vi "Dashboard Main.vi"() -> ()   [LabVIEW 2014]
uses:
  <vilib>/event_ctls.llb/eventvkey.ctl
  <vilib>/Rock Robotics/WPI/Dashboard/WPI_DashboardLogging Global.vi
  <vilib>/Utility/config.llb/Write Key (String).vi
  <vilib>/Utility/config.llb/Write Key (I32).vi
  <vilib>/Utility/config.llb/NI_LVConfig.lvlib
panel:
  in  "TCP":refnum<k5>
  in  "Rec Mode":enum32{"Stop", "Record", "Playback"}(radio)
  in  "Vision":u16(ring) items=["Camera Off", "USB Camera SW", "USB Camera HW", "IP Camera"]
  out "Camera IP":string
  out "Image Message":string="Timeout in Camera Communications"
  in  "Dashboard Tab":T1(tab)
  in  "Camera Settings":T2={"Frame Rate"=30, "Compression"=30, "Size"=1} {"Frame Rate" scale=1.0..30.0; "Size" items=["640x480", "320x240", "160x120"]}
  out "MotorChart R":cluster{"Numeric":dbl, "Numeric":dbl}(graph)
  out "MotorChart L":T3(graph)
  out "MotorSliders R":cluster{"MotorSlide1":dbl, "MotorSlide2":dbl} {"MotorSlide2" scale=-1.0..1.0 scale format="%#_2e"; "MotorSlide1" scale=-1.0..1.0 scale format="%#_2e"}
  out "MotorSliders L":T4 {"MotorSlide4 2" scale=0.0..14.0 scale format="%#_2e"; "MotorSlide2" scale=-1.0..1.0 scale format="%#_2e"; "MotorSlide1" scale=-1.0..1.0 scale format="%#_2e"}
  out "Gyro":dbl(knob) scale=0.0..360.0
  out "JS1 Z":dbl(slide) scale=-1.0..1.0 scale format="%#_2e"
  out "JS1 Graph":cluster{"X":dbl, "Y":dbl}[](graph)
  out "JS1 Buttons":T5
  out "JS2 Z":dbl(slide) scale=-1.0..1.0 scale format="%#_2e"
  out "JS2 Graph":cluster{"X":dbl, "Y":dbl}[](graph)
  out "JS2 Buttons":T5
  out "Mode":T6(ring)=enum."Auto Disabled"
  in  "DB Camera Config":bool
  out "fps":dbl format="%#.1g"
  out "Mbps":dbl format="%#.1g"
  out "Mbps 2":bool
  in  "DB/String 9":string
  in  "DB/String 8":string
  in  "DB/String 7":string
  in  "DB/String 6":string
  in  "DB/String 5":string
  in  "DB/String 4":string
  in  "DB/String 3":string
  in  "DB/String 2":string
  in  "DB/String 1":string
  in  "DB/String 0":string
  in  "DB/Slider 0":dbl(slide) scale=0.0..5.0
  in  "DB/Slider 1":dbl(slide) scale=0.0..5.0
  in  "DB/Slider 2":dbl(slide) scale=0.0..5.0
  in  "DB/Slider 3":dbl(slide) scale=0.0..5.0
  out "DB/LED 3":bool
  out "DB/LED 2":bool
  out "DB/LED 1":bool
  out "DB/LED 0":bool
  in  "DB/Button 3":bool
  in  "DB/Button 2":bool
  in  "DB/Button 1":bool
  in  "DB/Button 0":bool caption="New Name"
  in  "Test Slider":dbl(slide) scale=0.0..100.0 scale format="%#_3g"
  in  "On/Off":bool caption="Solenoid"
  in  "Test Name":u16(ring) items=["Select the test to run...", "Example Test", "-------------------------------", "List of tests is built in robot code.", "Replace with your own automated tests."]
  in  "Test Tree":string(tree)
  in  "Motor":cluster{"Value":dbl, "Enable":bool} {"Value" scale=-1.0..1.0 scale format="%#_3g"}
  out "Progress":T7 {"Test Progress" scale=0.0..100.0}
  in  "Rev/Fwd":cluster{"Forward":bool, "Reverse":bool}
  in  "Test Ring":u16(ring) items=["Monochrome", "Color"]
  in  "Listbox":i32(listbox)
  out "Tree":string(tree)
  out "Camera Image":T8(plugin-control)
  out "Boolean":bool
  # "Left"
  # "Front"
  # "Right"
  # "Battery"
  # "This tab is a great place for autonomous settings and robot-specific values.\nPlace controls and indicators inside this tab and match name to\nDashboard Variables on robot. You can also delete this comment."
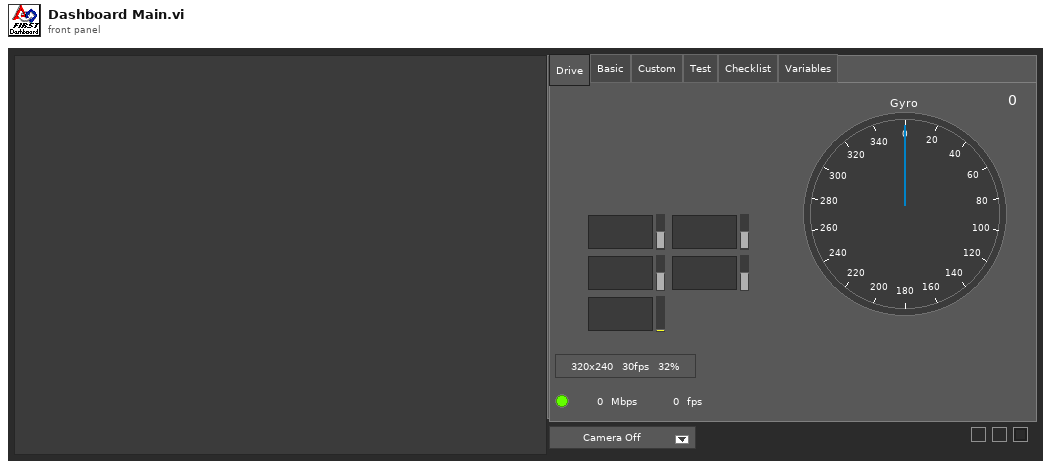
[diagram p1: front panel]
types:
  T1 = enum32{"Drive", "Basic", "Custom", "Test", "Checklist", "Variables"}
  T2 = cluster{"Frame Rate":i32, "Compression":i32, "Size":u16}
  T3 = cluster{"Numeric":dbl, "Numeric":dbl, "Battery V":dbl}
  T4 = cluster{"MotorSlide1":dbl, "MotorSlide2":dbl, "MotorSlide4 2":dbl}
  T5 = cluster{bool, bool, bool, bool, bool, bool, bool, bool, bool, bool, bool, bool}
  T6 = enum8{"Tele-Op Disabled", "Tele-Op Enabled", "Auto Disabled", "Auto Enabled", "Test Disabled", "Test Enabled", "Disconnected", "No Code", "E-Stop"}
  T7 = cluster{"Test Progress":u8, "Test Progress Text":string}
  T8 = typedef "IMAQ Image.ctl" = refnum<image>
  T9 = typedef "Image Type" = u32
  T10 = cluster{"Camera Image":refnum<vi>, "Dashboard Tab":refnum<vi>, "Boolean":refnum<vi>, "Vision":refnum<vi>, "Rec Mode":refnum<vi>, "Test Slider":refnum<vi>, "On/Off ":refnum<vi>, "Test Ring":refnum<vi>, "Rev/Fwd":refnum<vi>, "Test Name":refnum<vi>, "Motor":refnum<vi>, "Progress":refnum<vi>, "CheckList":refnum<vi>, "Tree":refnum<vi>, "Test Tree":refnum<vi>}
  T11 = cluster{"Error Strings":string, "Disable Counts":cluster{u16, u16}, "Rail Faults":cluster{u16, u16, u16}, "Robot IP":string, "DB Mode":u8, "Event Info":cluster{"Name":string, "Type":u8, "Number":u16, "Replay":u8}, "Camera Addr":string}
  T12 = cluster{"Storage":cluster{"Disk Free":u64, "RAM Block":u32, "RAM free":u32}, "CPU Utilization":cluster{"CPU % ISR":sgl, "CPU % Time Crit":sgl, "CPU % Timed Str":sgl, "CPU % High":sgl, "CPU % Above":sgl, "CPU % Normal":sgl, "CPU % Low":sgl}, "CAN":cluster{"% Bus Utilization":sgl, "Bus Off Cnt":u32, "TX_FIFO Full Cnt":u32, "Receive Error Cnt":u8, "Transmit Error Cnt":u8}, "HID":cluster{"HID Outputs":u32, "Rumble Low":u16, "Rumble High":u16}[]}
  T13 = cluster{"Status bits":cluster{"Test Mode":bool, "Autonomous":bool, "Enabled":bool, "Code Start":bool, "Brownout":bool, "Reserved 2":bool, "Reserved 3":bool, "E-Stop":bool}, "Code Trace":cluster{"Disabled":bool, "TeleOp":bool, "Auto":bool, "Test":bool}, "Controller Type":enum16{"unknown", "cRIO", "roboRio"}, "Code?":enum16{"unknown", "noCode", "code"}, "Battery V":dbl}
  T14 = cluster{"Control Bits":cluster{"TestMode":bool, "Autonomous":bool, "Enabled":bool, "FMS Present":bool, bool, bool, bool, "E-Stop":bool}, "Team Station ":u8, "Countdown":sgl, "Joystick Values":cluster{"Axes":dbl[], "Buttons":bool[], "POVs":i16[]}[]}
  T15 = cluster{"Axes":dbl[], "Buttons":bool[], "POVs":i16[]}[]
  T16 = cluster{"Axes":dbl[], "Buttons":bool[], "POVs":i16[]}
  T17 = cluster{"Buttons[0]":bool, "Buttons[1]":bool, "Buttons[2]":bool, "Buttons[3]":bool, "Buttons[4]":bool, "Buttons[5]":bool, "Buttons[6]":bool, "Buttons[7]":bool, "Buttons[8]":bool, "Buttons[9]":bool, "Buttons[10]":bool, "Buttons[11]":bool}
  T18 = typedef "NI_LVConfig.lvlib/Config Data RefNum.ctl" = refnum<k1>
  T19 = cluster{"Operation":enum16{"Update", "Clear"}, "Color Box":u32}[]
  T20 = typedef "eventvkey.ctl" = enum16{"ASCII", "Enter", "Return", "Shift", "Ctrl", "Alt", "Cmd", "Opt", "Caps", "NumLock", "Clear", "Break", "Up", "Down", "Left", "Right", "Insert", "Delete", "Home", "End", "PageUp", "PageDown", "Escape", "Help", "Pause", "ScrollLock", "F1", "F2", "F3", "F4", "F5", "F6", "F7", "F8", "F9", "F10", "F11", "F12", "F13", "F14", "F15", "F16", "F17", "F18", "F19", "F20", "F21", "F22", "F23", "F24", "Play", "VolumeUp", "VolumeDown", "Mute", "Two Byte Char"}
  T21 = cluster{"Image Size":bool, "Image Type":bool, "Pixel Value":bool, "ROI Information":bool, "Zoom Factor":bool}
  T22 = enum8{"Enabled", "Disabled", "Disabled and Grayed Out"}
  T23 = cluster{"Operation":enum16{"Update", "Clear"}, "Color Box":u32}
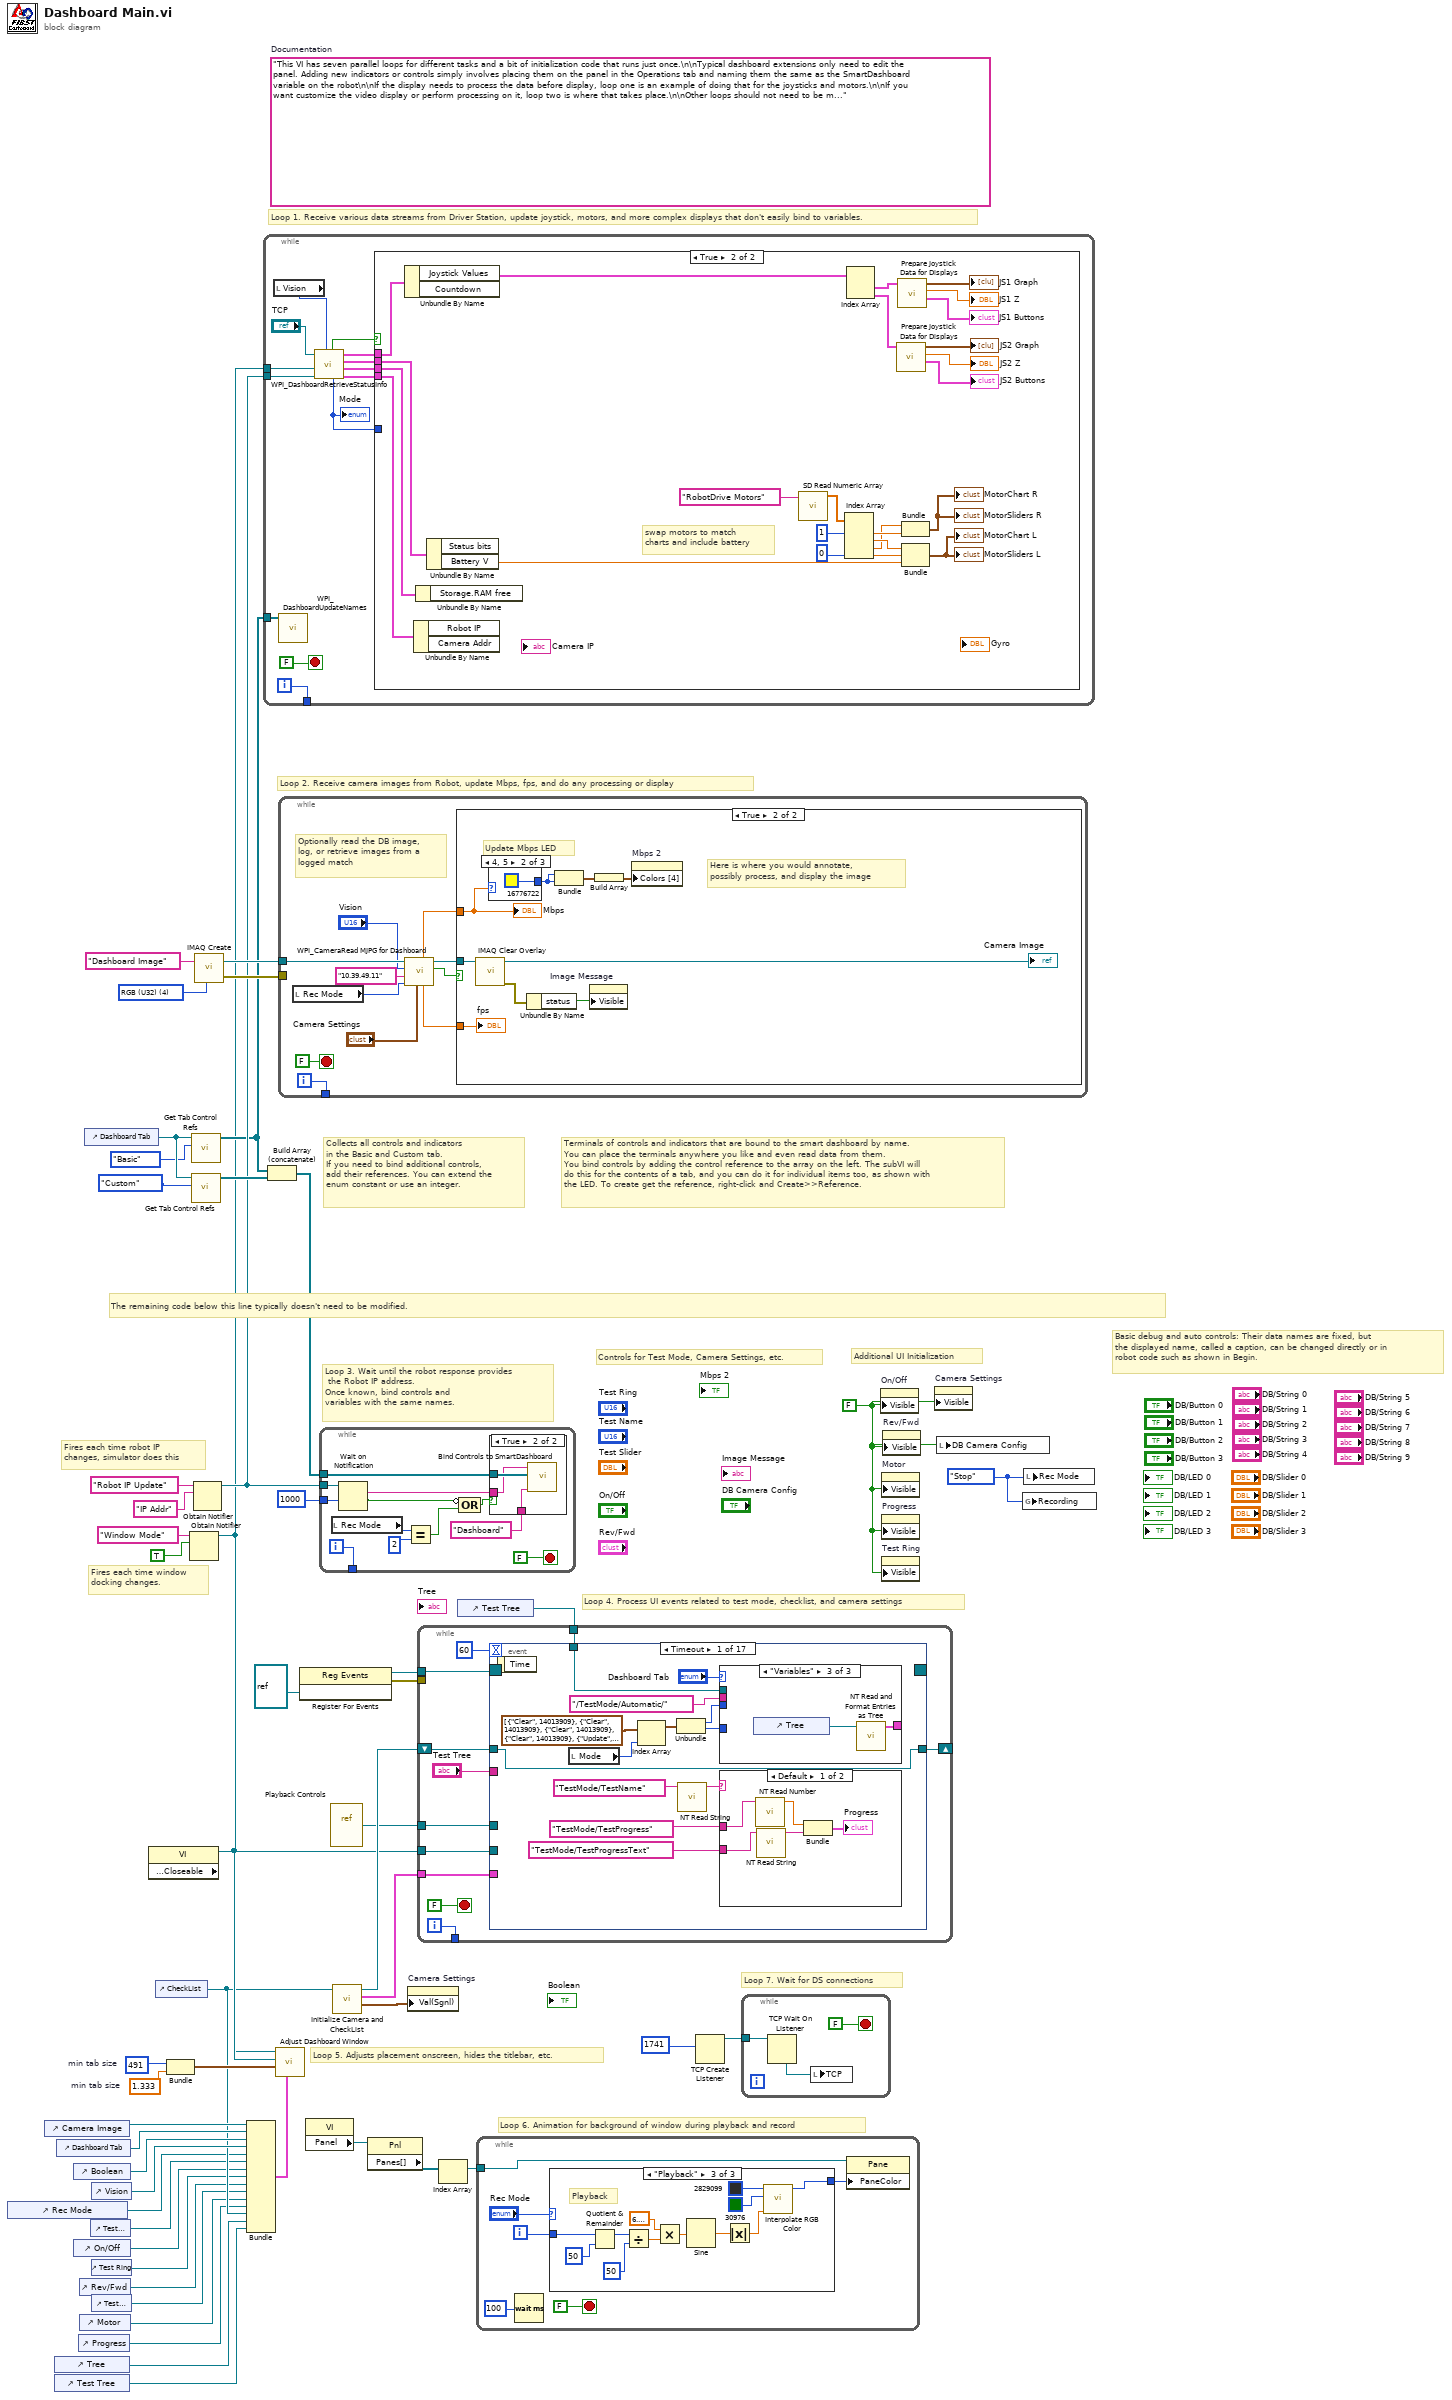
[diagram p0: block diagram]
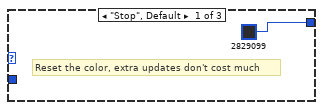
[diagram p3: hidden frame]
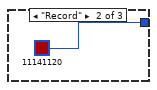
[diagram p4: hidden frame]
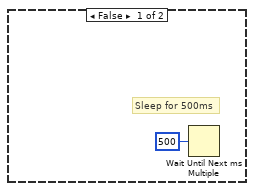
[diagram p6: hidden frame]
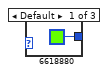
[diagram p7: hidden frame]
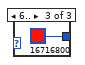
[diagram p8: hidden frame]
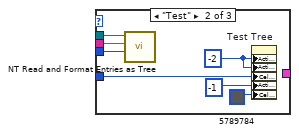
[diagram p10: hidden frame]
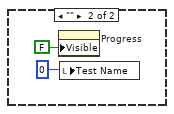
[diagram p11: hidden frame]
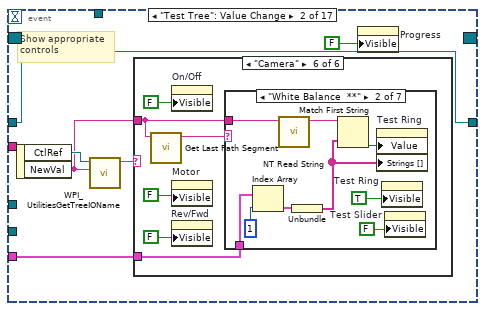
[diagram p12: hidden frame]
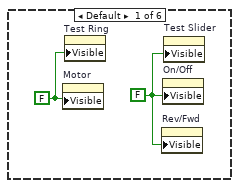
[diagram p13: hidden frame]
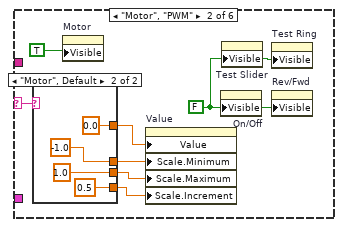
[diagram p14: hidden frame]
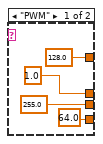
[diagram p15: hidden frame]
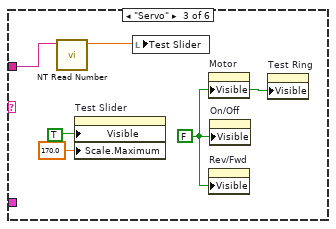
[diagram p16: hidden frame]
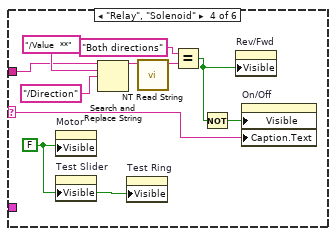
[diagram p17: hidden frame]
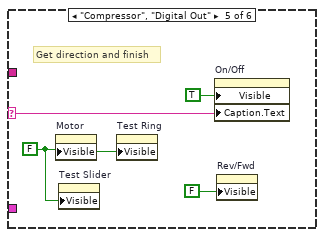
[diagram p18: hidden frame]
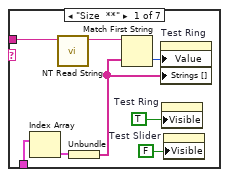
[diagram p19: hidden frame]
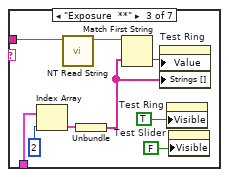
[diagram p20: hidden frame]
diagram:
  w24 = 491  # min tab size
  w23 = 1.333  # min tab size
  w32 = enum32{"Stop", "Record", "Playback"}."Stop" ("Rec Mode")
  w6 = FALSE ("Visible")
  (unwired) "This VI has seven parallel loops for different tasks and a bit of initialization code that runs just once.\n\nTypical dashboard extensions only need to edit the panel. Adding new indicators or controls simply involves placing them on the panel in the Operations tab and naming them the same as the SmartDashboard variable on the robot\n\nIf the display needs to process the data before display, loop one is an example of doing that for the joysticks and motors.\n\nIf you want customize the video display or perform processing on it, loop two is where that takes place.\n\nOther loops should not need to be modified. They are pretty standard, and document the task they perform."  # Documentation
  w52 = T9 4 items=["Grayscale (U8)", "Grayscale (I16)", "Grayscale (SGL)", "Complex (CSG)", "RGB (U32)", "HSL (U32)", "RGB (U64)"] ("Image Type")
  # "Loop 7. Wait for DS connections"
  # "Basic debug and auto controls: Their data names are fixed, but\nthe displayed name, called a caption, can be changed directly or in\nrobot code such as shown in Begin."
  # "Controls for Test Mode, Camera Settings, etc."
  # "Additional UI Initialization"
  # "Loop 6. Animation for background of window during playback and record"
  # "Fires each time robot IP\nchanges, simulator does this"
  # "Fires each time window\ndocking changes."
  # "Collects all controls and indicators\nin the Basic and Custom tab.\nIf you need to bind additional controls,\nadd their references. You can extend the\nenum constant or use an integer."
  # "The remaining code below this line typically doesn't need to be modified."
  # "Loop 4. Process UI events related to test mode, checklist, and camera settings"
  # "Terminals of controls and indicators that are bound to the smart dashboard by name.\nYou can place the terminals anywhere you like and even read data from them.\nYou bind controls by adding the control reference to the array on the left. The subVI will\ndo this for the contents of a tab, and you can do it for individual items too, as shown with\nthe LED. To create get the reference, right-click and Create>>Reference."
  # "Loop 3. Wait until the robot response provides\n the Robot IP address.\nOnce known, bind controls and\nvariables with the same names."
  # "Loop 5. Adjusts placement onscreen, hides the titlebar, etc."
  # "Loop 1. Receive various data streams from Driver Station, update joystick, motors, and more complex displays that don't easily bind to variables."
  # "Loop 2. Receive camera images from Robot, update Mbps, fps, and do any processing or display"
  n1 = control-ref of="Rec Mode"() -> (w12:refnum<vi>)
  n2 = control-ref of="Camera Image"() -> (w27:refnum<vi>)
  n3 = control-ref of="Tree"() -> (w16:refnum<vi>)
  n4 = control-ref of="Test Tree"() -> (w15:refnum<vi>)
  n5 = control-ref of="Dashboard Tab"() -> (w26:refnum<vi>)
  n6 = control-ref of="Boolean"() -> (w21:refnum<vi>)
  n7 = control-ref of="On/Off"() -> (w10:refnum<vi>)
  n8 = control-ref of="Progress"() -> (w7:refnum<vi>)
  n9 = control-ref of="Rev/Fwd"() -> (w8:refnum<vi>)
  n10 = control-ref of="Motor"() -> (w13:refnum<vi>)
  n11 = control-ref of="Dashboard Tab"() -> (w30:refnum<vi>)
  n12 = control-ref of="Test Slider"() -> (w11:refnum<vi>)
  n13 = control-ref of="Vision"() -> (w25:refnum<vi>)
  n14 = control-ref of="Test Ring"() -> (w9:refnum<vi>)
  n15 = control-ref of="Test Name"() -> (w14:refnum<vi>)
  n16 = property class="VI" props=["Front Panel.Closeable"]() -> (reference out=w31:refnum<vi>)  [unwired: 2 in, 2 out]
  n17 = control-ref of="CheckList"() -> (w17:refnum<vi>)
  n18 = Bundle("min tab size"=w24, "min tab size"=w23) -> (w22:cluster{"min tab size":i32, "min tab size":dbl})  [unwired: 1 in]
  n19 = Obtain Notifier(name (unnamed)="Window Mode", notification data type=TRUE) -> (notifier out=w3:refnum<notifier>)  [unwired: 2 in, 2 out]
  n20 = call <vilib>:"Get Tab Control Refs.vi"("Page Index"=T1."Basic" ("Dashboard Tab"), "TabControl in"=w30) -> ("ControlsOnPage"=w4:refnum<vi>[])  [unwired: 9 in]
  n21 = call <vilib>:"Get Tab Control Refs.vi"("Page Index"=T1."Custom" ("Dashboard Tab"), "TabControl in"=w30) -> ("ControlsOnPage"=w29:refnum<vi>[])  [unwired: 9 in]
  n22 = Obtain Notifier(name (unnamed)="Robot IP Update", notification data type="IP Addr" ("name (unnamed)")) -> (notifier out=w5:refnum<notifier>)  [unwired: 2 in, 2 out]
  n23 = call "IMAQ Create"("Image Name"="Dashboard Image", "Image Type"=w52) -> ("New Image"=w50:T8, "error out"=w49:errorcluster)  [unwired: 2 in, 1 out]
  n24 = Bundle("Camera Image"=w27, "Dashboard Tab"=w26, "Boolean"=w21, "Vision"=w25, "Rec Mode"=w12, "Test Slider"=w11, "On/Off"=w10, "Test Ring"=w9, "Rev/Fwd"=w8, "Test Name"=w14, "Motor"=w13, "Progress"=w7, "CheckList"=w17, "Tree"=w16, "Test Tree"=w15) -> (w18:T10)  [unwired: 1 in]
  n25 = while {
    tunnel: [w64] -> _
    tunnel: w5 -> [w58]
    tunnel: w4 -> [w57]
    tunnel: w3 -> [w53]
    i -> [w64]
    stop <- FALSE stop-if-true
    n26 = local read "Vision"() -> (w55:u16)
    n27 = call <vilib>:"WPI_DashboardUpdateNames.vi"("Controls on Tab"=w57) -> ()  [unwired: 11 in]
    n28 = call <vilib>:"WPI_DashboardRetrieveStatusInfo.vi"("Vision"=w55, "Binding Refnum"=w58, "Window Mode Notifier"=w53, "TCP Cnx"="TCP") -> ("Power and Errors"=w59:T11, "Robot Metrics"=w62:T12, "Status Info"=w63:T13, "Control Info"=w60:T14, "Robot Mode"=w56:T6, "Process?"=w61:bool)  [unwired: 2 in]
    "Mode" <- w56
    n29 = case shown="True" w61 {
      tunnel: w63 -> [_ w89]
      tunnel: w62 -> [_ w88]
      tunnel: w60 -> [_ w87]
      tunnel: w59 -> [_ w86]
      tunnel: w56 -> [_ _]
      frame False {
      }
      frame True {
        # "swap motors to match\ncharts and include battery"
        n30 = Unbundle By Name(w87) -> ("Joystick Values"=w74:T15)  [unwired: 1 out]
        n31 = Unbundle By Name(w86) -> ()  [unwired: 2 out]
        n32 = Unbundle By Name(w88) -> ()  [unwired: 1 out]
        n33 = Unbundle By Name(w89) -> ("Battery V"=w75:dbl)  [unwired: 1 out]
        n34 = call <vilib>:"SD Read Numeric Array.vi"("Name"="RobotDrive Motors") -> ("Numeric Array"=w77:dbl[])  [unwired: 8 in, 2 out]
        n35 = Index Array(array=w77, index #1=1, index #4=0) -> (element #1=w81:dbl, element #2=w82:dbl, element #3=w80:dbl, element #4=w85:dbl)  [unwired: 2 in]
        n36 = Index Array(array=w74) -> (element #1=w73:T16, element #2=w69:T16)  [unwired: 2 in]
        n37 = call "Prepare Joystick Data for Displays.vi"("Joystick Values"=w69) -> ("Buttons"=→"JS2 Buttons":T17, "Z Axis"=→"JS2 Z":dbl, "Cartesian Data"=→"JS2 Graph":cluster{"X axis":dbl, "X axis":dbl}[])  [unwired: 8 in]
        n38 = call "Prepare Joystick Data for Displays.vi"("Joystick Values"=w73) -> ("Buttons"=→"JS1 Buttons":T17, "Z Axis"=→"JS1 Z":dbl, "Cartesian Data"=→"JS1 Graph":cluster{"X axis":dbl, "X axis":dbl}[])  [unwired: 8 in]
        n39 = Bundle("Numeric"=w80, "Numeric"=w81) -> (→"MotorChart R" →"MotorSliders R":cluster{"Numeric":dbl, "Numeric":dbl})  [unwired: 1 in]
        n40 = Bundle("Numeric"=w82, "Numeric"=w85, "Battery V"=w75) -> (→"MotorChart L" →"MotorSliders L":T3)  [unwired: 1 in]
      }
    }
  }
  n41 = Build Array (concatenate)(w4, w29) -> (w28:refnum<vi>[])
  n42 = call "Adjust Dashboard Window.vi"("Sizing Refnums"=w18, "Size Constraints"=w22, "VI"=w31, "Notifier in"=w3) -> ()  [unwired: 8 in]
  n43 = while {
    tunnel: w50 -> [w98]
    tunnel: w49 -> [_]
    tunnel: [w99] -> _
    i -> [w99]
    stop <- FALSE stop-if-true
    # "Optionally read the DB image,\nlog, or retrieve images from a\nlogged match"
    n44 = local read "Rec Mode"() -> (w92:enum32{"Stop", "Record", "Playback"})
    n45 = call <vilib>:"WPI_CameraRead MJPG for Dashboard.vi"("Camera Settings"="Camera Settings", "Rec Mode"=w92, "Camera IP"="10.39.49.11", "Camera Mode"="Vision", "Refnum in"=w98) -> ("Active"=w96:bool, "Refnum out"=w97:T8, "FPS"=w95:dbl, "Bandwidth (Mbps)"=w94:dbl)  [unwired: 3 in]
    n46 = case shown="True" w96 {
      tunnel: w97 -> [_ w105]
      tunnel: w94 -> [_ w104]
      tunnel: w95 -> [_ w102]
      frame False {
        # "Sleep for 500ms"
        n47 = Wait Until Next ms Multiple(millisecond multiple=u32 500) -> ()  [unwired: 1 out]
      }
      frame True {
        # "Here is where you would annotate,\npossibly process, and display the image"
        # "Update Mbps LED"
        n48 = call "IMAQ Clear Overlay"("Image"=w105) -> ("error out"=w109:errorcluster, "Image Out"=→"Camera Image":T8)  [unwired: 2 in, 7 out]
        n49 = case shown="4, 5" w104 {
          tunnel: [u32 6618880 ("Color Box") u32 16776722 ("Color Box") u32 16716800 ("Color Box")] -> w106
          frame Default {
          }
          frame 4, 5 {
          }
          frame 6.. {
          }
        }
        n50 = Unbundle By Name(w109) -> ("status"=w110:bool)
        n51 = Bundle("Color Box"=w106, "Color Box"=w106) -> (w108:cluster{"Color Box":u32, "Color Box":u32})  [unwired: 1 out]
        n52 = property on="Image Message" class="Str"("Visible"=w110) -> ()  [unwired: 2 in, 2 out]
        n53 = Build Array(w108) -> (w107:cluster{"Color Box":u32, "Color Box":u32}[])
        n54 = property on="Mbps 2" class="Bool (strict)"("Colors [4]"=w107) -> ()  [unwired: 2 in, 2 out]
        "Mbps" <- w104
        "fps" <- w102
      }
    }
  }
  n55 = register-events(refnum<vi> refnum) -> (reference out=w36:refnum<event-registration>, error out=w35:errorcluster)  [unwired: 2 in]
  n56 = property class="VI"() -> ("Panel"=w39:refnum<vi>)  [unwired: 2 in, 2 out]
  n57 = while {
    tunnel: w28 -> [w125]
    tunnel: w5 -> [w123]
    tunnel: [w121] -> _
    tunnel: u32 1000 ("milliseconds to wait") -> [w120]
    i -> [w121]
    stop <- FALSE stop-if-true
    n58 = local read "Rec Mode"() -> (w116:enum32{"Stop", "Record", "Playback"})
    n59 = Wait on Notification(notifier=w123, timeout in ms (-1)=w120) -> (notification=w122:string, timed out?=w118:bool)  [unwired: 2 in, 2 out]
    n60 = Equal?(x=w116, y=u16 2 ("Rec Mode")) -> (x = y?=w117:bool)
    n61 = Compound Arithmetic op=OR(invert w118, w117) -> (w119:bool)
    n62 = case shown="True" w119 {
      tunnel: w125 -> [_ w128]
      tunnel: w122 -> [_ w127]
      tunnel: "Dashboard" -> [_ w126]
      frame False {
      }
      frame True {
        n63 = call <vilib>:"Bind Controls to SmartDashboard.vi"("Client Name"=w126, "Bound Control Refs"=w128, "Server IP Address"=w127) -> ()  [unwired: 9 in]
      }
    }
  }
  n64 = vi-ref "Playback Controls.vi"() -> (w37:refnum<vi>)
  n65 = call "Initialize Camera and CheckList.vi"("ListBox in"=w17) -> ("Cluster"=w43:cluster{"value":i32, "value":i32, "index":i32}, "Array"=w44:cluster{string[]}[], "File Refnum"=w42:T18)  [unwired: 8 in]
  n66 = property class="Pnl"(reference=w39) -> ("Panes[]"=w40:refnum<vi>[])  [unwired: 1 in, 2 out]
  n67 = property on="Camera Settings" class="Clust (strict)"("Val(Sgnl)"=w43) -> ()  [unwired: 2 in, 2 out]
  n68 = Index Array(array=w40) -> (element=w38:refnum<vi>)  [unwired: 1 in]
  n69 = control-ref of="Test Tree"() -> (w41:refnum<vi>)
  n70 = while {
    tunnel: w44 -> [w136]
    shift-right: [w135] -> _
    shift-left: w42 -> [w134]
    tunnel: [w133] -> _
    tunnel: w41 -> [w132]
    tunnel: w37 -> [w131]
    tunnel: w36 -> [w130]
    tunnel: w35 -> [_]
    tunnel: w31 -> [w129]
    i -> [w133]
    stop <- FALSE stop-if-true
    n71 = event shown="[0] Timeout" {
      selector: w130 -> [_ _ _ _ _ _ _ _ _ _ _ _ _ _ _ _ _]
      dyn-events: [_ _ _ _ _ _ _ _ _ _ _ _ _ w374 _ _ _] -> _
      timeout: u32 60 ("milliseconds to wait") -> [_ _ _ _ _ _ _ _ _ _ _ _ _ _ _ _ _]
      tunnel: w132 -> [w148 _ _ _ _ _ _ _ _ _ _ _ _ _ _ _ _]
      tunnel: "Test Tree" -> [_ _ _ _ _ _ _ _ w343 w351 w353 w357 w365 _ _ _ _]
      tunnel: w136 -> [_ w170 _ _ _ _ w307 w337 _ _ _ _ _ _ _ _ _]
      tunnel: [w144 w169 w268 w273 w281 w293 w306 w330 w342 w349 w352 w356 w364 w376 w390 w391 w401] -> w135
      tunnel: w134 -> [w144 w169 w268 w273 w281 w293 w305 w330 w342 w349 w352 w356 w364 w376 w390 w391 w401]
      tunnel: w131 -> [_ _ _ _ _ _ _ _ _ _ _ _ _ w377 _ w394 _]
      tunnel: w129 -> [_ _ _ _ _ _ _ _ _ _ _ _ _ w372 _ _ _]
      event Timeout {
        n72 = event-data() -> ()  [unwired: 1 in, 1 out]
        n73 = local read "Mode"() -> (w147:T6)
        n74 = Index Array(array=T19 [{"Operation"=enum."Clear", "Color Box"=14013909}, {"Operation"=enum."Clear", "Color Box"=14013909}, {"Operation"=enum."Clear", "Color Box"=14013909}, {"Operation"=enum."Clear", "Color Box"=14013909}, {"Operation"=enum."Update", "Color Box"=14013909}, {"Operation"=enum."Update", "Color Box"=16777215}, {"Operation"=enum."Clear", "Color Box"=14013909}, {"Operation"=enum."Clear", "Color Box"=14013909}, {"Operation"=enum."Clear", "Color Box"=14013909}], index=w147) -> (element=w142:T23)
        n75 = Unbundle(w142) -> ("Operation"=w141:enum16{"Update", "Clear"}, "Color Box"=w140:u32)
        n76 = call <vilib>:"NT Read String.vi"("Name"="TestMode/TestName") -> ("String"=w151:string)  [unwired: 9 in, 1 out]
        n77 = case shown="\"Variables\"" "Dashboard Tab" {
          tunnel: w148 -> [_ w159 _]
          tunnel: "/TestMode/Automatic/" ("Name Pattern") -> [_ w158 _]
          tunnel: w141 -> [_ w157 _]
          tunnel: [_ _ w161] -> _
          tunnel: w140 -> [_ w153 _]
          frame "Custom", Default {
          }
          frame "Test" {
            w156 = -2 ("Active Item:Row Number")
            n78 = call <vilib>:"NT Read and Format Entries as Tree.vi"("Operation"=w157, "Name Pattern"=w158, "Tree Refnum"=w159) -> ()  [unwired: 7 in, 2 out]
            n79 = property on="Test Tree" class="Tree (strict)"("Active Item Row Number"=w156, "ActiveColNum"=w156, "CellBG"=w153, "Active Item Row Number"=-1 ("Active Item:Row Number"), "CellBG"=u32 5789784 ("Color Box")) -> ()  [unwired: 2 in, 2 out]
          }
          frame "Variables" {
            n80 = control-ref of="Tree"() -> (w160:refnum<vi>)
            n81 = call <vilib>:"NT Read and Format Entries as Tree.vi"("Tree Refnum"=w160) -> ("Formatted Strings"=w161:cluster{"Name":string, "Value":string}[])  [unwired: 9 in, 1 out]
          }
        }
        n82 = case shown="Default" w151 {
          tunnel: "TestMode/TestProgress" ("Name") -> [w163 _]
          tunnel: "TestMode/TestProgressText" ("Name") -> [w162 _]
          frame Default {
            n83 = call <vilib>:"NT Read Number.vi"("Name"=w163) -> ("Numeric"=w164:dbl)  [unwired: 9 in, 1 out]
            n84 = call <vilib>:"NT Read String.vi"("Name"=w162) -> ("String"=w165:string)  [unwired: 9 in, 1 out]
            n85 = Bundle("Numeric"=w164, "String"=w165) -> (→"Progress":cluster{"Numeric":dbl, "String":string})  [unwired: 1 in]
          }
          frame "" {
            n86 = property on="Progress" class="Clust (strict)"("Visible"=FALSE) -> ()  [unwired: 2 in, 2 out]
            n87 = local write "Test Name"(u16 0) -> ()
          }
        }
      }
      event "Test Tree": Value Change {
        # "Show appropriate\ncontrols"
        n88 = event-data() -> ("CtlRef"=w173:refnum<vi>, "NewVal"=w171:string)  [unwired: 1 in]
        n89 = call <vilib>:"WPI_UtilitiesGetTreeIOName.vi"("NewVal"=w171, "TreeControl in"=w173) -> ("I/O Name"=w174:string)  [unwired: 9 in]
        n90 = case shown="\"Camera\"" w174 {
          selector: w174 -> [_ w181 _ w199 w208 _]
          tunnel: w171 -> [_ _ w196 w198 _ w215]
          tunnel: w170 -> [_ _ _ _ _ w214]
          frame Default {
            w176 = FALSE ("Visible")
            w175 = FALSE ("Visible")
            n91 = property on="Motor" class="Clust (strict)"("Visible"=w175) -> ()  [unwired: 2 in, 2 out]
            n92 = property on="Test Ring" class="Ring (strict)"("Visible"=w175) -> ()  [unwired: 2 in, 2 out]
            n93 = property on="Rev/Fwd" class="Clust (strict)"("Visible"=w176) -> ()  [unwired: 2 in, 2 out]
            n94 = property on="On/Off" class="Bool (strict)"("Visible"=w176) -> ()  [unwired: 2 in, 2 out]
            n95 = property on="Test Slider" class="Slide (strict)"("Visible"=w176) -> ()  [unwired: 2 in, 2 out]
          }
          frame "Motor", "PWM" {
            w182 = FALSE ("Visible")
            n96 = case shown="\"Motor\", Default" w181 {
              tunnel: [1.0 ("Value") -1.0 ("Value")] -> w180
              tunnel: [255.0 ("Value") 1.0 ("Value")] -> w179
              tunnel: [128.0 ("Value") 0.0 ("Value")] -> w178
              tunnel: [64.0 ("Value") 0.5 ("Value")] -> w177
              frame "PWM" {
              }
              frame "Motor", Default {
              }
            }
            n97 = property on="Motor" class="Clust (strict)"("Visible"=TRUE) -> ()  [unwired: 2 in, 2 out]
            n98 = property on="Value" class="Slide (strict)"("Value"=w178, "Scale.Minimum"=w180, "Scale.Maximum"=w179, "Scale.Increment"=w177) -> ()  [unwired: 2 in, 2 out]
            n99 = property on="On/Off" class="Bool (strict)"("Visible"=w182) -> ()  [unwired: 2 in, 2 out]
            n100 = property on="Test Slider" class="Slide (strict)"("Visible"=w182) -> ()  [unwired: 2 in, 2 out]
            n101 = property on="Test Ring" class="Ring (strict)"("Visible"=w182) -> ()  [unwired: 2 in, 2 out]
            n102 = property on="Rev/Fwd" class="Clust (strict)"("Visible"=w182) -> ()  [unwired: 2 in, 2 out]
          }
          frame "Servo" {
            w194 = FALSE ("Visible")
            n103 = call <vilib>:"NT Read Number.vi"("Name"=w196) -> ("Numeric"=w195:dbl)  [unwired: 9 in, 1 out]
            n104 = property on="Test Slider" class="Slide (strict)"("Visible"=TRUE, "Scale.Maximum"=170.0 ("Scale.Range:Maximum")) -> ()  [unwired: 2 in, 2 out]
            n105 = local write "Test Slider"(w195) -> ()
            n106 = property on="Motor" class="Clust (strict)"("Visible"=w194) -> ()  [unwired: 2 in, 2 out]
            n107 = property on="Rev/Fwd" class="Clust (strict)"("Visible"=w194) -> ()  [unwired: 2 in, 2 out]
            n108 = property on="On/Off" class="Bool (strict)"("Visible"=w194) -> ()  [unwired: 2 in, 2 out]
            n109 = property on="Test Ring" class="Ring (strict)"("Visible"=w194) -> ()  [unwired: 2 in, 2 out]
          }
          frame "Relay", "Solenoid" {
            w197 = FALSE ("Visible")
            n110 = property on="Motor" class="Clust (strict)"("Visible"=w197) -> ()  [unwired: 2 in, 2 out]
            n111 = property on="Test Slider" class="Slide (strict)"("Visible"=w197) -> ()  [unwired: 2 in, 2 out]
            n112 = Search and Replace String(input string=w198, search string="/Value  **", replace string="/Direction") -> (result string=w204:string)  [unwired: 5 in, 3 out]
            n113 = property on="Test Ring" class="Ring (strict)"("Visible"=w197) -> ()  [unwired: 2 in, 2 out]
            n114 = call <vilib>:"NT Read String.vi"("Name"=w204) -> ("String"=w202:string)  [unwired: 9 in, 1 out]
            n115 = Equal?(x="Both directions", y=w202) -> (x = y?=w200:bool)
            n116 = Not(x=w200) -> (.not. x?=w201:bool)
            n117 = property on="Rev/Fwd" class="Clust (strict)"("Visible"=w200) -> ()  [unwired: 2 in, 2 out]
            n118 = property on="On/Off" class="Bool (strict)"("Visible"=w201, "Caption.Text"=w199) -> ()  [unwired: 2 in, 2 out]
          }
          frame "Compressor", "Digital Out" {
            w207 = FALSE ("Visible")
            # "Get direction and finish"
            n119 = property on="Motor" class="Clust (strict)"("Visible"=w207) -> ()  [unwired: 2 in, 2 out]
            n120 = property on="Test Slider" class="Slide (strict)"("Visible"=w207) -> ()  [unwired: 2 in, 2 out]
            n121 = property on="Test Ring" class="Ring (strict)"("Visible"=w207) -> ()  [unwired: 2 in, 2 out]
            n122 = property on="On/Off" class="Bool (strict)"("Visible"=TRUE, "Caption.Text"=w208) -> ()  [unwired: 2 in, 2 out]
            n123 = property on="Rev/Fwd" class="Clust (strict)"("Visible"=FALSE) -> ()  [unwired: 2 in, 2 out]
          }
          frame "Camera" {
            n124 = call <vilib>:"Get Last Path Segment.vi"("String in"=w215) -> ("String out"=w216:string)  [unwired: 10 in]
            n125 = property on="On/Off" class="Bool (strict)"("Visible"=FALSE) -> ()  [unwired: 2 in, 2 out]
            n126 = property on="Motor" class="Clust (strict)"("Visible"=FALSE) -> ()  [unwired: 2 in, 2 out]
            n127 = property on="Rev/Fwd" class="Clust (strict)"("Visible"=FALSE) -> ()  [unwired: 2 in, 2 out]
            n128 = case shown="\"White Balance  **\"" w216 {
              tunnel: w215 -> [w222 w231 w240 w249 w258 _ w264]
              tunnel: w214 -> [w220 w228 w237 w246 w255 _ _]
              frame "Size  **" {
                n129 = Index Array(array=w220) -> (element=w219:cluster{string[]})  [unwired: 1 in]
                n130 = call <vilib>:"NT Read String.vi"("Name"=w222) -> ("String"=w221:string)  [unwired: 9 in, 1 out]
                n131 = Unbundle(w219) -> (w217:string[])
                n132 = Match First String(2:w217, 3:w221) -> (0:w218:i32)  [unwired: 1 out]
                n133 = property on="Test Ring" class="Ring (strict)"("Value"=w218, "Strings []"=w217) -> ()  [unwired: 2 in, 2 out]
                n134 = property on="Test Ring" class="Ring (strict)"("Visible"=TRUE) -> ()  [unwired: 2 in, 2 out]
                n135 = property on="Test Slider" class="Slide (strict)"("Visible"=FALSE) -> ()  [unwired: 2 in, 2 out]
              }
              frame "White Balance  **" {
                n136 = Index Array(array=w228, index=1) -> (element=w229:cluster{string[]})
                n137 = call <vilib>:"NT Read String.vi"("Name"=w231) -> ("String"=w230:string)  [unwired: 9 in, 1 out]
                n138 = Unbundle(w229) -> (w226:string[])
                n139 = Match First String(2:w226, 3:w230) -> (0:w225:i32)  [unwired: 1 out]
                n140 = property on="Test Ring" class="Ring (strict)"("Value"=w225, "Strings []"=w226) -> ()  [unwired: 2 in, 2 out]
                n141 = property on="Test Ring" class="Ring (strict)"("Visible"=TRUE) -> ()  [unwired: 2 in, 2 out]
                n142 = property on="Test Slider" class="Slide (strict)"("Visible"=FALSE) -> ()  [unwired: 2 in, 2 out]
              }
              frame "Exposure  **" {
                n143 = Index Array(array=w237, index=2) -> (element=w238:cluster{string[]})
                n144 = call <vilib>:"NT Read String.vi"("Name"=w240) -> ("String"=w239:string)  [unwired: 9 in, 1 out]
                n145 = Unbundle(w238) -> (w234:string[])
                n146 = Match First String(2:w234, 3:w239) -> (0:w235:i32)  [unwired: 1 out]
                n147 = property on="Test Ring" class="Ring (strict)"("Value"=w235, "Strings []"=w234) -> ()  [unwired: 2 in, 2 out]
                n148 = property on="Test Ring" class="Ring (strict)"("Visible"=TRUE) -> ()  [unwired: 2 in, 2 out]
                n149 = property on="Test Slider" class="Slide (strict)"("Visible"=FALSE) -> ()  [unwired: 2 in, 2 out]
              }
              frame "Exposure Priority  **" {
                n150 = Index Array(array=w246, index=3) -> (element=w247:cluster{string[]})
                n151 = call <vilib>:"NT Read String.vi"("Name"=w249) -> ("String"=w248:string)  [unwired: 9 in, 1 out]
                n152 = Unbundle(w247) -> (w243:string[])
                n153 = Match First String(2:w243, 3:w248) -> (0:w244:i32)  [unwired: 1 out]
                n154 = property on="Test Ring" class="Ring (strict)"("Value"=w244, "Strings []"=w243) -> ()  [unwired: 2 in, 2 out]
                n155 = property on="Test Ring" class="Ring (strict)"("Visible"=TRUE) -> ()  [unwired: 2 in, 2 out]
                n156 = property on="Test Slider" class="Slide (strict)"("Visible"=FALSE) -> ()  [unwired: 2 in, 2 out]
              }
              frame "Color Enable  **" {
                n157 = Index Array(array=w255, index=4) -> (element=w256:cluster{string[]})
                n158 = call <vilib>:"NT Read String.vi"("Name"=w258) -> ("String"=w257:string)  [unwired: 9 in, 1 out]
                n159 = Unbundle(w256) -> (w252:string[])
                n160 = Match First String(2:w252, 3:w257) -> (0:w253:i32)  [unwired: 1 out]
                n161 = property on="Test Ring" class="Ring (strict)"("Value"=w253, "Strings []"=w252) -> ()  [unwired: 2 in, 2 out]
                n162 = property on="Test Ring" class="Ring (strict)"("Visible"=TRUE) -> ()  [unwired: 2 in, 2 out]
                n163 = property on="Test Slider" class="Slide (strict)"("Visible"=FALSE) -> ()  [unwired: 2 in, 2 out]
              }
              frame Default {
                n164 = property on="Test Ring" class="Ring (strict)"("Visible"=FALSE) -> ()  [unwired: 2 in, 2 out]
                n165 = property on="Test Slider" class="Slide (strict)"("Visible"=FALSE) -> ()  [unwired: 2 in, 2 out]
              }
              frame "Brightness  **", "Color Level  **", "Compression  **", "FPS  **", "Sharpness  **" {
                n166 = call <vilib>:"NT Read Number.vi"("Name"=w264) -> ("Numeric"=w263:dbl)  [unwired: 9 in, 1 out]
                n167 = local write "Test Slider"(w263) -> ()
                n168 = property on="Test Slider" class="Slide (strict)"("Visible"=TRUE, "Scale.Maximum"=100.0 ("Scale.Range:Maximum")) -> ()  [unwired: 2 in, 2 out]
                n169 = property on="Test Ring" class="Ring (strict)"("Visible"=FALSE) -> ()  [unwired: 2 in, 2 out]
              }
            }
          }
        }
        n170 = property on="Progress" class="Clust (strict)"("Visible"=FALSE) -> ()  [unwired: 2 in, 2 out]
      }
      event "Test Name": Mouse Enter {
        # "Populate the ring with the list of tests"
        n171 = event-data() -> ()  [unwired: 1 in, 1 out]
        n172 = call <vilib>:"NT Read String Array.vi"("Name"="TestMode/TestList") -> ("String Array"=w272:string[])  [unwired: 9 in, 1 out]
        n173 = Build Array (concatenate)("Select the test to run...", w272) -> (w271:string[])
        n174 = property on="Test Name" class="Ring (strict)"("Strings []"=w271) -> ()  [unwired: 2 in, 2 out]
      }
      event "Test Name": Value Change {
        w274 = FALSE ("Visible")
        # "Tell the robot the test name to run"
        n175 = event-data() -> ("NewVal"=w278:u16)  [unwired: 1 in]
        n176 = property on="Test Name" class="Ring (strict)"() -> ("Strings []"=w279:string[])  [unwired: 2 in, 2 out]
        n177 = local write "Progress"(T7 {"Test Progress"=0, "Test Progress Text"=""} ("Progress")) -> ()
        n178 = Index Array(array=w279, index=w278) -> (element=w277:string)
        n179 = call <vilib>:"NT Write String.vi"("String"=w277, "Name"="TestMode/TestName") -> ()  [unwired: 9 in, 1 out]
        n180 = property on="Progress" class="Clust (strict)"("Visible"=TRUE) -> ()  [unwired: 2 in, 2 out]
        n181 = property on="Motor" class="Clust (strict)"("Visible"=w274) -> ()  [unwired: 2 in, 2 out]
        n182 = property on="Test Slider" class="Slide (strict)"("Visible"=w274) -> ()  [unwired: 2 in, 2 out]
        n183 = property on="On/Off" class="Bool (strict)"("Visible"=w274) -> ()  [unwired: 2 in, 2 out]
        n184 = property on="Rev/Fwd" class="Clust (strict)"("Visible"=w274) -> ()  [unwired: 2 in, 2 out]
        n185 = property on="Test Ring" class="Ring (strict)"("Visible"=w274) -> ()  [unwired: 2 in, 2 out]
      }
      event "Listbox": Double Click {
        # "Shift clears all"
        # "Update symbols on the listbox"
        n186 = event-data() -> ("PlatMods.Shift"=w282:bool, "Row"=w284:i32)  [unwired: 1 in]
        n187 = case shown="True" w282 {
          tunnel: w284 -> [w288 _]
          tunnel: 1 -> [w287 _]
          frame False {
            n188 = property on="Listbox" class="LstBox (strict)"() -> ("Item Symbols"=w286:i32[])  [unwired: 2 in, 2 out]
            n189 = Replace Array Subset(array=w286, new element=w287, index=w288) -> (w285:i32[])
            n190 = property on="Listbox" class="LstBox (strict)"("Item Symbols"=w285) -> ()  [unwired: 2 in, 2 out]
          }
          frame True {
            w289 = 0 ("Top Row")
            n191 = property on="Listbox" class="LstBox (strict)"() -> ("Number of Rows"=w291:u32)  [unwired: 2 in, 2 out]
            n192 = Initialize Array(0, w291) -> (w290:i32[])
            n193 = property on="Listbox" class="LstBox (strict)"("Top Row"=w289, "Value"=w289, "Item Symbols"=w290) -> ()  [unwired: 2 in, 2 out]
          }
        }
      }
      event "Listbox": Key Down {
        # "Update symbols on the listbox\nLeft and right keys check and uncheck"
        n194 = event-data() -> ("VKey"=w295:T20)  [unwired: 1 in]
        n195 = case shown="\"Left\", \"Right\"" w295 {
          selector: w295 -> [w300 _]
          tunnel: eventvkey."Left" ("VKey") -> [w298 _]
          frame "Left", "Right" {
            n196 = Equal?(x=w298, y=w300) -> (x = y?=w299:bool)
            n197 = Select(t=0, s=w299, f=1) -> (s? t:f=w301:i32)
            n198 = property on="Listbox" class="LstBox (strict)"() -> ("Item Symbols"=w304:i32[])  [unwired: 2 in, 2 out]
            n199 = Replace Array Subset(array=w304, new element=w301, index="Listbox") -> (w303:i32[])
            n200 = property on="Listbox" class="LstBox (strict)"("Item Symbols"=w303) -> ()  [unwired: 2 in, 2 out]
          }
          frame Default {
          }
        }
      }
      event "DB Camera Config": Value Change {
        # "Show or hide the cluster of controls, store in ini file"
        n201 = event-data() -> ("NewVal"=w308:bool)  [unwired: 1 in]
        n202 = case shown="False" w308 {
          tunnel: w307 -> [w317 _]
          tunnel: [w310 w328] -> w306
          tunnel: w305 -> [w309 w328]
          frame False {
            w324 = "Camera"
            w327 = FALSE ("Visible")
            n203 = local read "Camera Settings"() -> (w316:T2)
            n204 = Index Array(array=w317) -> (element=w320:cluster{string[]})  [unwired: 1 in]
            n205 = Unbundle(w316) -> ("Frame Rate"=w315:i32, "Compression"=w314:i32, "Size"=w318:u16)
            n206 = Unbundle(w320) -> (w319:string[])
            n207 = Index Array(array=w319, index=w318) -> (element=w313:string)
            n208 = call-poly <vilib>:"Write Key.vi"("section"=w324, "value"=w313, "key"="Size", "refnum"=w309) -> ("refnum out"=w326:T18)  [unwired: 2 in, 5 out]
            n209 = call-poly <vilib>:"Write Key.vi"("section"=w324, "value"=w315, "key"="FrameRate", "refnum"=w326) -> ("refnum out"=w325:T18)  [unwired: 1 in, 6 out]
            n210 = property on="Camera Settings" class="Clust (strict)"("Visible"=w327) -> ()  [unwired: 2 in, 2 out]
            n211 = local write "DB Camera Config"(w327) -> ()
            n212 = call-poly <vilib>:"Write Key.vi"("section"=w324, "value"=w314, "key"="Compression", "refnum"=w325) -> ("refnum out"=w311:T18)  [unwired: 1 in, 6 out]
            n213 = call <vilib>:"Close Config Data.vi"("refnum"=w311) -> ("file path"=w312:path)  [unwired: 2 in, 8 out]
            n214 = call <vilib>:"Open Config Data.vi"("configuration file path"=w312) -> ("refnum"=w310:T18)  [unwired: 8 in, 2 out]
          }
          frame True {
            n215 = property on="Camera Settings" class="Clust (strict)"("Visible"=TRUE) -> ()  [unwired: 2 in, 2 out]
          }
        }
      }
      event "Camera Settings": Value Change {
        # "Update summary string when any elements of DB camera change"
        n216 = event-data() -> ("NewVal"=w341:T2)  [unwired: 1 in]
        n217 = Index Array(array=w337) -> (element=w336:cluster{string[]})  [unwired: 1 in]
        n218 = Unbundle(w341) -> ("Frame Rate"=w332:i32, "Compression"=w331:i32, "Size"=w334:u16)
        n219 = Unbundle(w336) -> (w335:string[])
        n220 = Index Array(array=w335, index=w334) -> (element=w333:string)
        n221 = Format Into String(format string="%s   %dfps   %d%%", w333, w332, w331) -> (resulting string=w338:string)  [unwired: 2 in, 1 out]
        n222 = Build Array(w338) -> (w339:string[])
        n223 = property on="DB Camera Config" class="Bool (strict)"("Strings [4]"=w339) -> ()  [unwired: 2 in, 2 out]
      }
      event "Motor.Enable": Value Change {
        # "When the test mode otor enable helper is set, update that\ntree row item's value"
        n224 = event-data() -> ("NewVal"=w347:bool)  [unwired: 1 in]
        n225 = Unbundle("Motor") -> ("Value"=w346:dbl)  [unwired: 1 out]
        n226 = Select(t=w346, s=w347, f=0.0) -> (s? t:f=w344:dbl)
        n227 = call <vilib>:"NT Write Number.vi"("Numeric"=w344, "Name"=w343) -> ()  [unwired: 9 in, 1 out]
      }
      event "Test Slider": Value Change {
        # "When the test mode slider helper is set, update that\ntree row item's value"
        n228 = event-data() -> ("NewVal"=w350:dbl)  [unwired: 1 in]
        n229 = call <vilib>:"NT Write Number.vi"("Numeric"=w350, "Name"=w351) -> ()  [unwired: 9 in, 1 out]
      }
      event "On/Off": Value Change {
        # "When the test mode on/off helper value is set, update that\ntree row item's value"
        n230 = event-data() -> ("NewVal"=w355:bool)  [unwired: 1 in]
        n231 = Boolean To (0,1)(Boolean=w355) -> (0, 1=w354:i16)
        n232 = call <vilib>:"NT Write Number.vi"("Numeric"=w354, "Name"=w353) -> ()  [unwired: 9 in, 1 out]
      }
      event "Rev/Fwd": Value Change {
        # "When the test mode helper value for relays is set, update that\ntree row item's value"
        n233 = event-data() -> ("NewVal.Forward"=w363:bool, "NewVal.Reverse"=w362:bool)  [unwired: 1 in]
        n234 = Boolean To (0,1)(Boolean=w363) -> (0, 1=w359:i16)
        n235 = Boolean To (0,1)(Boolean=w362) -> (0, 1=w361:i16)
        n236 = Negate(x=w361) -> (-x=w360:i16)
        n237 = Add(x=w359, y=w360) -> (x+y=w358:i16)
        n238 = call <vilib>:"NT Write Number.vi"("Numeric"=w358, "Name"=w357) -> ()  [unwired: 9 in, 1 out]
      }
      event "Test Ring": Value Change {
        # "When a test mode helper value is selected from the ring,\nset the tree item's variable to the string value"
        n239 = event-data() -> ("NewVal"=w367:u16)  [unwired: 1 in]
        n240 = property on="Test Ring" class="Ring (strict)"() -> ("Strings []"=w368:string[])  [unwired: 2 in, 2 out]
        n241 = Index Array(array=w368, index=w367) -> (element=w366:string)
        n242 = call <vilib>:"NT Write String.vi"("String"=w366, "Name"=w365) -> ()  [unwired: 9 in, 1 out]
      }
      event "Rec Mode": Value Change {
        # "Update globals for recording mode and path to read log from.\nClear when logging and let NetworkTables set path for vision to\nuse."
        n243 = event-data() -> ("NewVal"=w378:enum32{"Stop", "Record", "Playback"})  [unwired: 1 in]
        n244 = global write "WPI_DashboardLogging Global.vi" "Logging Filename"(path "") -> ()
        n245 = case shown="\"Playback\"" w378 {
          tunnel: w377 -> [_ w380 w388]
          tunnel: [_ _ w387] -> w374
          tunnel: [_ _ w386] -> _
          tunnel: w372 -> [_ _ w384]
          tunnel: cluster{i32, i32} {-250, 170} -> [_ _ w383]
          tunnel: [_ _ T21 {"Image Size"=TRUE, "Image Type"=TRUE, "Pixel Value"=TRUE, "ROI Information"=TRUE, "Zoom Factor"=FALSE} ("Image Information Shown:All Elements")] -> w370
          tunnel: [_ _ TRUE ("Zoom Factor")] -> w369
          frame Default {
          }
          frame "Stop", "Record" {
            # "Place Window too"
            n246 = invoke class="VI" method="FP.Close"(reference=w380) -> (reference out=w379:refnum<vi>)  [unwired: 2 in, 2 out]
            n247 = invoke class="VI" method="Abort VI"(reference=w379) -> ()  [unwired: 2 in, 3 out]
          }
          frame "Playback" {
            n248 = call "Open Playback Panel.vi"("Offset"=w383, "DB VI Ref"=w384, "Playback in"=w388) -> ("Playback out"=w385:refnum<vi>)  [unwired: 8 in]
            n249 = register-events(w385) -> (reference out=w387:refnum<event-registration>, error out=w386:errorcluster)  [unwired: 2 in]
          }
        }
        n250 = global write "WPI_DashboardLogging Global.vi" "Recording"(w378) -> ()
        n251 = property on="Camera Image" class="ImageControl"("Image Information Shown"=w370, "Image Information Visible"=w369) -> ()  [unwired: 2 in, 2 out]
        n252 = call <vilib>:"WPI_DashboardNT Log FieldName Cache.vi"("Operation"=enum16{"Lookup/Add", "Index", "Clear"}."Clear") -> ()  [unwired: 8 in, 3 out]
      }
      event Panel Close {
        w389 = enum32{"Stop", "Record", "Playback"}."Stop" ("Rec Mode")
        # "Playback window has been closed, abort"
        n253 = event-data() -> ()  [unwired: 1 in, 4 out]
        n254 = local write "Rec Mode"(w389) -> ()
        n255 = global write "WPI_DashboardLogging Global.vi" "Recording"(w389) -> ()
      }
      event Panel Close {
        # "Abort playback window and ourself"
        n256 = event-data() -> ()  [unwired: 1 in, 4 out]
        n257 = invoke class="VI" method="FP.Close"(reference=w394) -> (reference out=w393:refnum<vi>)  [unwired: 2 in, 2 out]
        n258 = invoke class="VI" method="Abort VI"(reference=w393) -> (error out=w392:errorcluster)  [unwired: 2 in, 2 out]
        n259 = invoke class="VI" method="Abort VI"(error in=w392) -> ()  [unwired: 2 in, 3 out]
      }
      event "Vision": Value Change {
        # "Enable/Disable Compression slider.\nHW USB is hard-coded into the camera"
        n260 = event-data() -> ("NewVal"=w400:u16)  [unwired: 1 in]
        n261 = Equal?(x=w400, y=u32 2 ("milliseconds to wait")) -> (x = y?=w398:bool)
        n262 = Select(t=T22."Disabled and Grayed Out" ("Disabled"), s=w398, f=T22."Enabled" ("Disabled")) -> (s? t:f=w395:T22)
        n263 = property on="Compression" class="Slide (strict)"("DisabledEnum"=w395) -> ()  [unwired: 2 in, 2 out]
      }
    }
  }
  n264 = while {
    tunnel: w38 -> [w403]
    i -> [w406]
    stop <- FALSE stop-if-true
    n265 = Wait (ms)(milliseconds to wait=u32 100) -> ()  [unwired: 1 out]
    n266 = case shown="\"Playback\"" "Rec Mode" {
      tunnel: w406 -> [_ _ w421]
      tunnel: [u32 2829099 ("Base Color") u32 11141120 ("Target Color") w410] -> w402
      frame "Stop", Default {
        # "Reset the color, extra updates don't cost much"
      }
      frame "Record" {
      }
      frame "Playback" {
        # "Playback"
        n267 = Quotient & Remainder(x=w421, y=u32 50 ("milliseconds to wait")) -> (x-y*floor(x/y)=w417:u32)  [unwired: 1 out]
        n268 = Divide(x=w417, y=u32 50 ("milliseconds to wait")) -> (x/y=w414:dbl)
        n269 = Multiply(x=6.283185307179586, y=w414) -> (x*y=w419:dbl)
        n270 = Sine(x=w419) -> (sin(x)=w418:dbl)
        n271 = Absolute Value(x=w418) -> (abs(x)=w411:dbl)
        n272 = call "Interpolate RGB Color.vi"("Proportion"=w411, "Target Color"=u32 30976, "Base Color"=u32 2829099) -> ("Result Color"=w410:u32)  [unwired: 8 in]
      }
    }
    n273 = property class="Pane"(reference=w403, "PaneColor"=w402) -> ()  [unwired: 1 in, 2 out]
  }
  n274 = TCP Create Listener(10:u16 1741 ("timeout ms (25000)")) -> (3:w1:refnum<k5>)  [unwired: 4 in, 2 out]
  n275 = while {
    tunnel: w1 -> [w423]
    stop <- FALSE stop-if-true
    n276 = TCP Wait On Listener(11:w423) -> (4:w422:refnum<k5>)  [unwired: 3 in, 4 out]
    n277 = local write "TCP"(w422) -> ()
  }
  n278 = property on="On/Off" class="Bool (strict)"("Visible"=w6) -> ()  [unwired: 2 in, 2 out]
  n279 = property on="Motor" class="Clust (strict)"("Visible"=w6) -> ()  [unwired: 2 in, 2 out]
  n280 = property on="Progress" class="Clust (strict)"("Visible"=w6) -> ()  [unwired: 2 in, 2 out]
  n281 = property on="Test Ring" class="Ring (strict)"("Visible"=w6) -> ()  [unwired: 2 in, 2 out]
  n282 = property on="Rev/Fwd" class="Clust (strict)"("Visible"=w6) -> ()  [unwired: 2 in, 2 out]
  n283 = property on="Camera Settings" class="Clust (strict)"("Visible"=w6) -> ()  [unwired: 2 in, 2 out]
  n284 = local write "DB Camera Config"(w6) -> ()
  n285 = global write "WPI_DashboardLogging Global.vi" "Recording"(w32) -> ()
  n286 = local write "Rec Mode"(w32) -> ()
